vi "Set ATP ComboBox - Multiple Projects Open.vi"(8 "Error In":errorcluster, 9 "User VI Filepath":path, 10 "Project Refs":refnum<vi>[](array[refnum]), 11 "Project Name ComboBox Ref":refnum<vi>) -> (0 "Error Out":errorcluster)   [LabVIEW 2022 SP3]
doc: "ATP = \"Add to Project?\" drop-down menu"
uses:
  <vilib>/Utility/miscctls.llb/LVFontTypeDef.ctl
panel:
  out "Value":string
  out "Strings[]":string[](array[string])
  out "Distances":i32[](array[numeric])
  out "Iteration":i32
  # "Development\nControls or indicators that are useful for development or testing, but which are not outputs of the VI."
  # "Input\nInputs to the VI"
  # "Output\nOutputs of the VI"
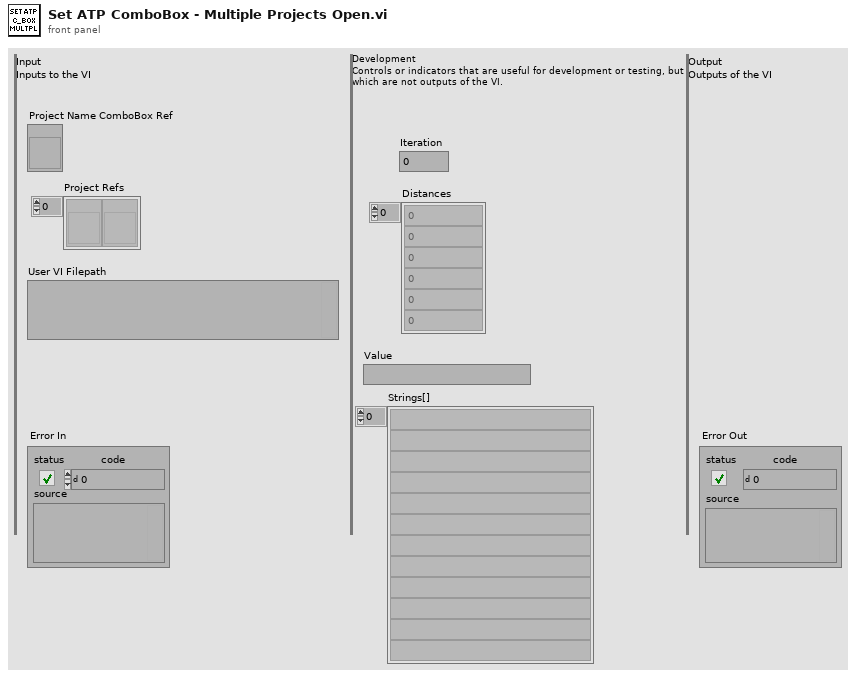
[diagram p1: front panel]
types:
  T1 = typedef "LVFontTypeDef.ctl" = cluster{"Font Name":string, "Size":u16, "Bold":bool, "Italic":bool, "Underline":bool, "Strikeout":bool, "Color":u32}
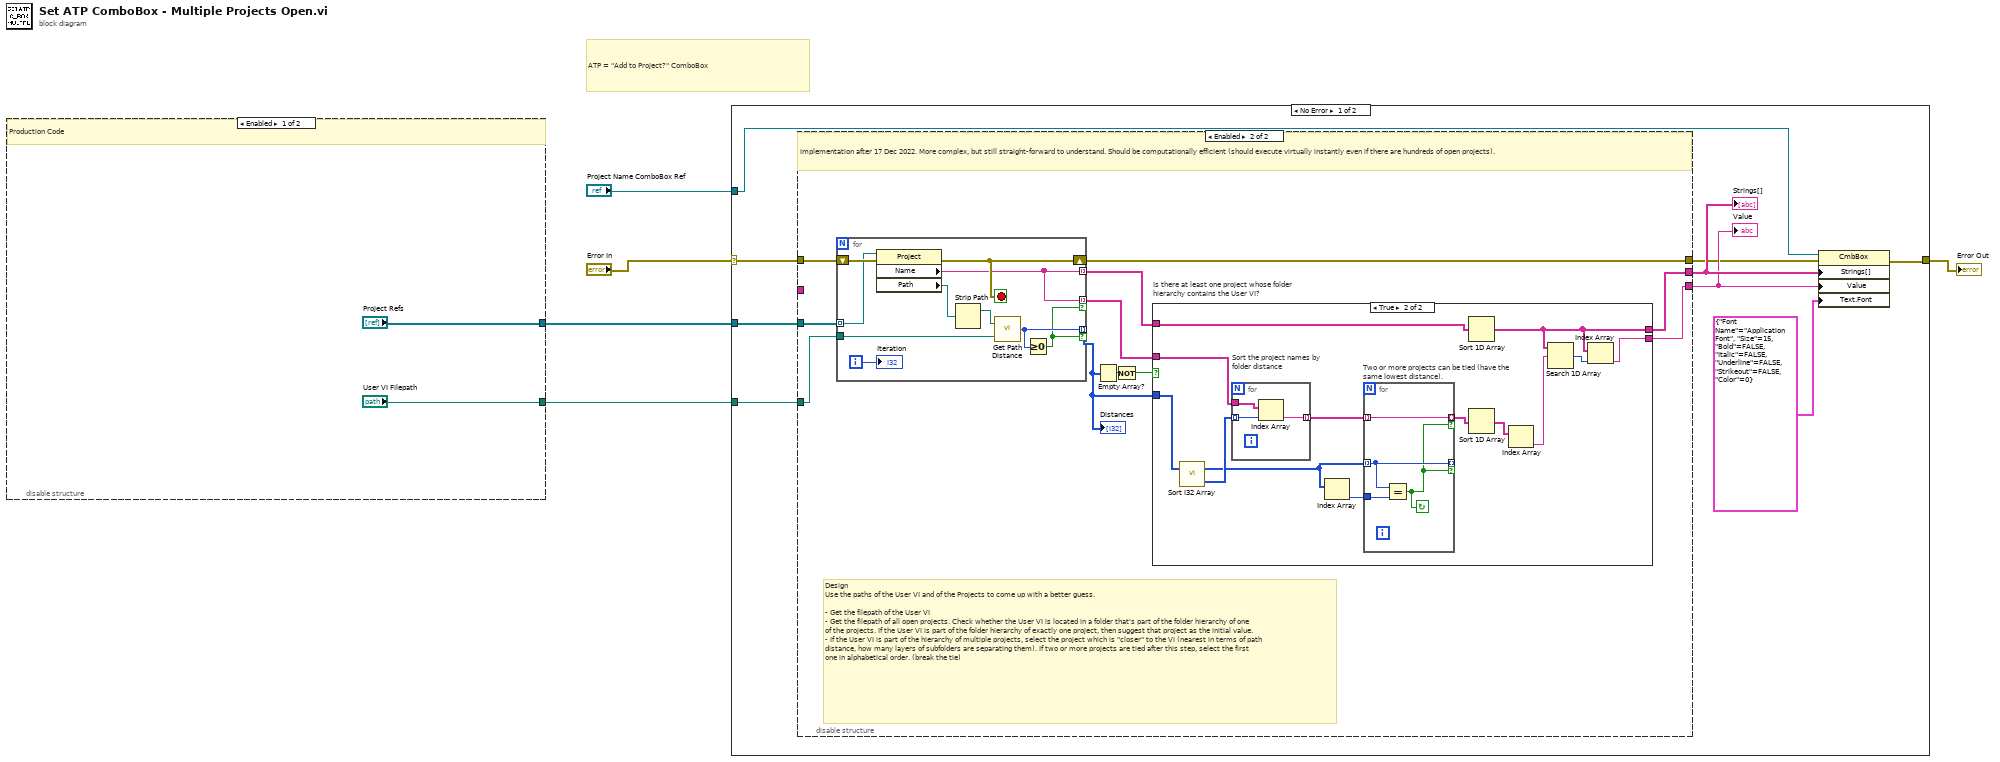
[diagram p0: block diagram]
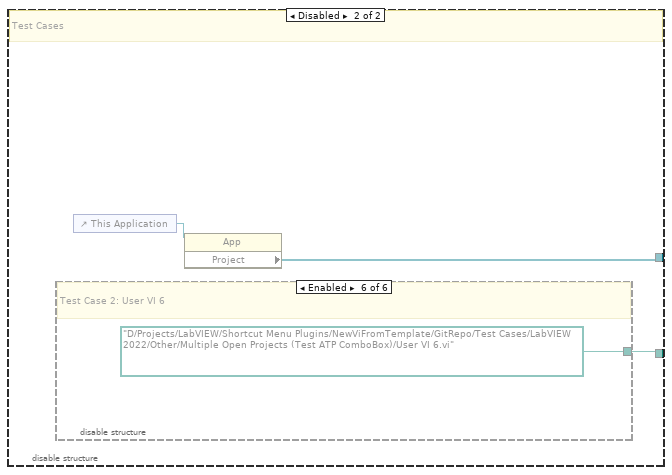
[diagram p2: hidden frame]
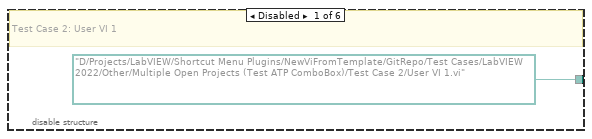
[diagram p3: hidden frame]
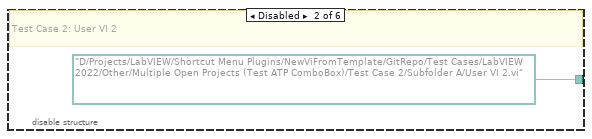
[diagram p4: hidden frame]
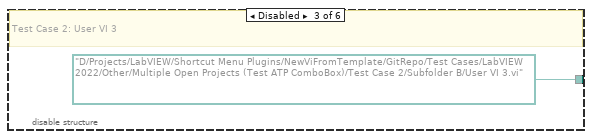
[diagram p5: hidden frame]
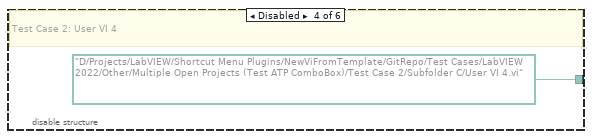
[diagram p6: hidden frame]
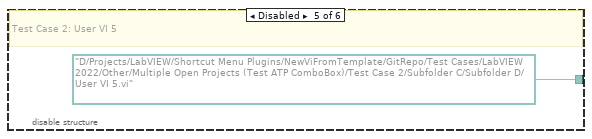
[diagram p7: hidden frame]
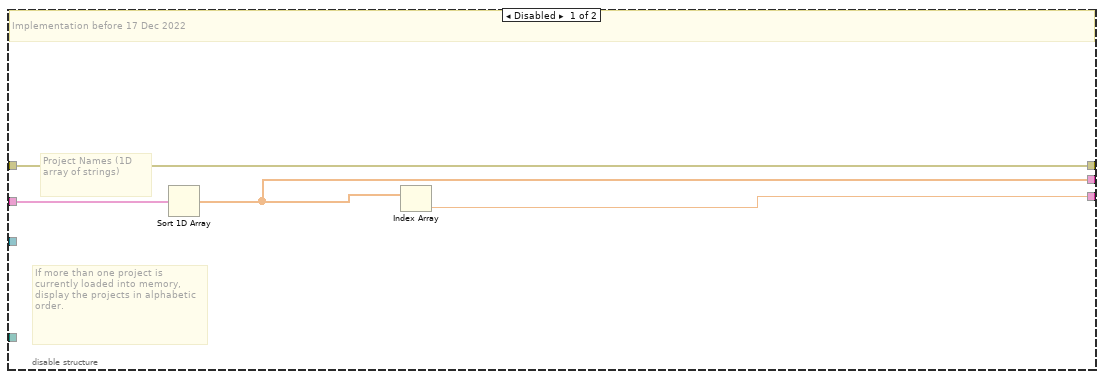
[diagram p8: hidden frame]
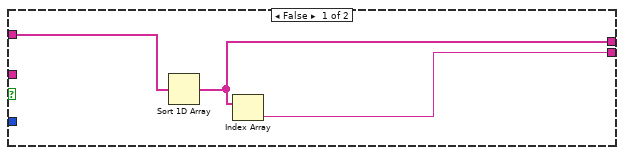
[diagram p9: hidden frame]
diagram:
  # "ATP = \"Add to Project?\" ComboBox"
  n1 = disable-structure shown="Enabled" {
    disable-tunnel: ["Project Refs" w8] -> w2
    disable-tunnel: ["User VI Filepath" w10] -> w1
    frame Enabled {
      # "Production Code"
    }
    frame Disabled {
      # "Test Cases"
      n2 = disable-structure shown="Enabled" {
        disable-tunnel: [path "D:/Projects/LabVIEW/Shortcut Menu Plugins/NewViFromTemplate/GitRepo/Test Cases/LabVIEW 2022/Other/Multiple Open Projects (Test ATP ComboBox)/Test Case 2/User VI 1.vi" path "D:/Projects/LabVIEW/Shortcut Menu Plugins/NewViFromTemplate/GitRepo/Test Cases/LabVIEW 2022/Other/Multiple Open Projects (Test ATP ComboBox)/Test Case 2/Subfolder A/User VI 2.vi" path "D:/Projects/LabVIEW/Shortcut Menu Plugins/NewViFromTemplate/GitRepo/Test Cases/LabVIEW 2022/Other/Multiple Open Projects (Test ATP ComboBox)/Test Case 2/Subfolder B/User VI 3.vi" path "D:/Projects/LabVIEW/Shortcut Menu Plugins/NewViFromTemplate/GitRepo/Test Cases/LabVIEW 2022/Other/Multiple Open Projects (Test ATP ComboBox)/Test Case 2/Subfolder C/User VI 4.vi" path "D:/Projects/LabVIEW/Shortcut Menu Plugins/NewViFromTemplate/GitRepo/Test Cases/LabVIEW 2022/Other/Multiple Open Projects (Test ATP ComboBox)/Test Case 2/Subfolder C/Subfolder D/User VI 5.vi" path "D:/Projects/LabVIEW/Shortcut Menu Plugins/NewViFromTemplate/GitRepo/Test Cases/LabVIEW 2022/Other/Multiple Open Projects (Test ATP ComboBox)/User VI 6.vi"] -> w10
        frame Disabled {
          # "Test Case 2: User VI 1"
        }
        frame Disabled {
          # "Test Case 2: User VI 2"
        }
        frame Disabled {
          # "Test Case 2: User VI 3"
        }
        frame Disabled {
          # "Test Case 2: User VI 4"
        }
        frame Disabled {
          # "Test Case 2: User VI 5"
        }
        frame Enabled {
          # "Test Case 2: User VI 6"
        }
      }
      n3 = control-ref of="This Application"() -> (w9:refnum<vi>)
      n4 = property class="App"(reference=w9) -> ("Project"=w8:refnum<vi>[])  [unwired: 1 in, 2 out]
    }
  }
  n5 = case shown="No Error" "Error In" {
    selector: "Error In" -> [w20 w74]
    tunnel: [w22 w74] -> w4
    tunnel: "Project Name ComboBox Ref" -> [w25 _]
    tunnel: w2 -> [w18 _]
    tunnel: w1 -> [w17 _]
    frame No Error {
      n6 = disable-structure shown="Enabled" {
        disable-tunnel: _ -> [w29 _]
        disable-tunnel: [w28 w32] -> w24
        disable-tunnel: [w27 w31] -> w23
        disable-tunnel: w20 -> [w26 w40]
        disable-tunnel: [w26 w39] -> w19
        disable-tunnel: w18 -> [_ w38]
        disable-tunnel: w17 -> [_ w37]
        frame Disabled {
          # "Project Names (1D array of strings)"
          # "If more than one project is currently loaded into memory, display the projects in alphabetic order."
          # "Implementation before 17 Dec 2022"
          n7 = Sort 1D Array(array=w29) -> (sorted array=w28:ext[])
          n8 = Index Array(array=w28) -> (element=w27:ext)  [unwired: 1 in]
        }
        frame Enabled {
          # "Design\nUse the paths of the User VI and of the Projects to come up with a better guess.\n\n- Get the filepath of the User VI\n- Get the filepath of all open projects. Check whether the User VI is located in a folder that's part of the folder hierarchy of one of the projects. If the User VI is part of the folder hierarchy of exactly one project, then suggest that project as the initial value.\n- If the User VI is part of the hierarchy of multiple projects, select the project which is \"closer\" to the VI (nearest in terms of path distance, how many layers of subfolders are separating them). If two or more projects are tied after this step, select the first one in alphabetical order. (break the tie)"
          # "Implementation after 17 Dec 2022. More complex, but still straight-forward to understand. Should be computationally efficient (should execute virtually instantly even if there are hundreds of open projects)."
          n9 = for {
            shift-right: [w71] -> w39
            shift-left: w40 -> [w73]
            tunnel: w38 -> [w72] mode=indexing
            tunnel: [w65] -> w36 mode=indexing
            tunnel: w37 -> [w67]
            tunnel: [w66] -> w35 mode=indexing if=w64
            tunnel: [w65] -> w30 mode=indexing if=w64
            i -> [w70]
            stop <- w71 stop-if-true
            n10 = property class="Project"(reference=w72, error in=w73) -> (error out=w71:errorcluster, "Name"=w65:string, "Path"=w69:path)  [unwired: 1 out]
            n11 = Strip Path(path=w69) -> (stripped path=w68:path)  [unwired: 1 out]
            n12 = call "Get Path Distance.vi"("Filepath"=w67, "Folder Path"=w68) -> ("Distance"=w66:i32)
            n13 = Greater Or Equal To 0?(x=w66) -> (x >= 0?=w64:bool)
            "Iteration" <- w70
          }
          "Distances" <- w35
          n14 = Empty Array?(array=w35) -> (empty?=w34:bool)
          n15 = Not(x=w34) -> (.not. x?=w33:bool)
          n16 = case "Is there at least one project whose folder hierarchy contains the User VI?" shown="True" w33 {
            tunnel: w35 -> [_ w56]
            tunnel: w36 -> [w43 w44]
            tunnel: [w42 w45] -> w32
            tunnel: [w41 w48] -> w31
            tunnel: w30 -> [_ w53]
            frame False {
              n17 = Sort 1D Array(array=w43) -> (sorted array=w42:string[])
              n18 = Index Array(array=w42) -> (element=w41:string)  [unwired: 1 in]
            }
            frame True {
              n19 = call "Sort I32 Array.vi"("Array in"=w56) -> ("Sorted Pointers"=w55:i32[], "Sorted Array out"=w47:i32[])  [unwired: 1 in]
              n20 = for "Sort the project names by\nfolder distance" {
                tunnel: w53 -> [w63]
                tunnel: w55 -> [w62] mode=indexing
                tunnel: [w61] -> w52 mode=indexing
                n21 = Index Array(array=w63, index=w62) -> (element=w61:string)
              }
              n22 = Index Array(array=w47) -> (element=w54:i32)  [unwired: 1 in]
              n23 = for "Two or more projects can be tied (have the same lowest distance)." {
                tunnel: w47 -> [w59] mode=indexing
                tunnel: w54 -> [w60]
                tunnel: w52 -> [w58] mode=indexing
                tunnel: [w59] -> _ mode=indexing if=w57
                tunnel: [w58] -> w51 mode=indexing if=w57
                stop <- w57 continue-if-true
                n24 = Equal?(x=w59, y=w60) -> (x = y?=w57:bool)
              }
              n25 = Sort 1D Array(array=w44) -> (sorted array=w45:string[])
              n26 = Sort 1D Array(array=w51) -> (sorted array=w46:string[])
              n27 = Index Array(array=w46) -> (element=w50:string)  [unwired: 1 in]
              n28 = Search 1D Array(1D array=w45, element=w50) -> (index of element=w49:i32)  [unwired: 1 in]
              n29 = Index Array(array=w45, index=w49) -> (element=w48:string)
            }
          }
        }
      }
      "Strings[]" <- w24
      "Value" <- w23
      n30 = property class="CmbBox"(reference=w25, error in=w19, "Strings[]"=w24, "Value"=w23, "Text.Font"=T1 {"Font Name"="Application Font", "Size"=15, "Bold"=FALSE, "Italic"=FALSE, "Underline"=FALSE, "Strikeout"=FALSE, "Color"=0}) -> (error out=w22:errorcluster)  [unwired: 1 out]
    }
    frame Error {
    }
  }
  "Error Out" <- w4
